vi "Empty Cluster.vi"() -> (0 "Empty Cluster":variant)   [LabVIEW 2020, in "JKI JSON Serialization.lvlib"]
uses:
  JKI JSON Serialization.lvlib
  <userlib>/_OpenG.lib/lvdata/lvdata.llb/openg_variant.lvlib
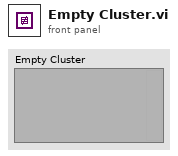
[diagram p1: front panel]
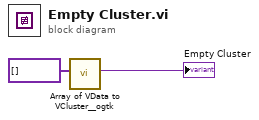
[diagram p0: block diagram]
diagram:
  n1 = call <userlib>:"Array of VData to VCluster__ogtk.vi"("Array"=variant[] []) -> ("VCluster"=→"Empty Cluster":variant)  [unwired: 9 in, 1 out]
